vi "myRIO_BRig_RT__Case_Exp_State_SelectPre__v4.vi"(0 "input_dataCurrent":u16[](array[numeric]), 1 "input_SelectWrong":bool, 2 "input_SelectReward":bool, 5 "input_dataExp":u16[](array[numeric]), 7 "input_LickL":bool, 9 "input_LickR":bool, 11 "input_arrTrig":bool[](array[boolean])) -> (3 "output_state":T1, 4 "output_dataCurrent":u16[](array[numeric]), 8 "output_l1_laserEvent":bool, 10 "output_l1_laserOn":bool, 13 "output_l2_laserOn":bool, 14 "output_l2_laserEvent":bool)   [LabVIEW 2014]
uses:
  myRIO_BRig_RT__Case_Exp_stateList.ctl
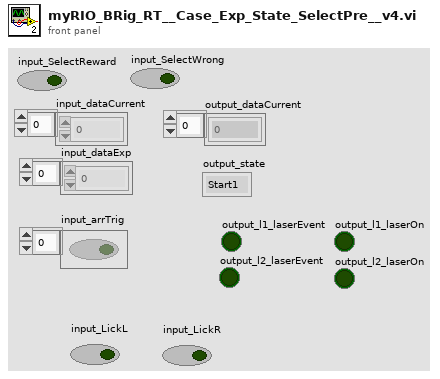
[diagram p1: front panel]
types:
  T1 = typedef "myRIO_BRig_RT__Case_Exp_stateList.ctl" = enum16{"Start1", "Start2", "Start3", "saveSettings1", "saveSettings2", "saveSettings3", "saveSettings4", "saveSettings_LC_ENL_l1", "saveSettings_LC_ENL_l2", "saveSettings_LC_Cue_l1", "saveSettings_LC_Cue_l2", "saveSettings6_LC_l1_Other", "SaveSettings6_LC_l2_Other", "setSettings_Audio", "setSettings_Laser", "initBlock_pre", "initBlock", "initBlock2", "initBlock_post", "initTrial_pre", "initTrial", "initTrial2", "initTrial3", "initTrial4", "initTrial_LC_ENL1", "initTrial_LC_Cue1", "initTrial_LC_Cue1_2", "initTrial_LC_Sel", "initTrial_post", "ENL1_pre", "ENL1", "ENL1_post", "ENL1Penalty_pre", "ENL1Penalty", "ENL2_pre", "ENL2", "ENL2Penalty_pre", "ENL2Penalty", "Cue1_pre", "Cue1", "Cue1_post", "Cue1Penalty_pre", "Cue1Penalty", "Cue2_pre", "Cue2", "Cue2Penalty_pre", "Cue2Penalty", "Selection_pre", "Selection", "Select_post", "SelectReward_pre", "SelectReward", "SelectRewardPost_pre", "SelectRewardPost", "SelectWrong_pre", "SelectWrong", "SelectWrong_post", "SelectTimeout_pre", "SelectTimeout", "SelectTimeout_post", "endTrial_pre", "endTrial1", "endTrial2", "endTrial3", "endTrial_post", "endBlock_pre", "endBlock", "endBlock_post", "endExp", "commConnect", "commUpload_pre", "commUpload_dataBlock", "commUpload_dataCurrent", "commUpload_dataExp", "commUpload_dataLC", "commUpload_dataTrial", "commUpload_post", "saveData_pre", "saveData_dataBlock", "saveData_dataCurrent", "saveData_dataExp", "saveData_dataLC", "saveData_dataTrial", "saveData_post", "empty_endBlock1", "empty_endBlock2", "empty_endTrial1", "empty_endTrial2", "empty_endTrial3", "empty_endTrial4", "empty_endTrial5", "dummyState", "dummyState_endBlock"}
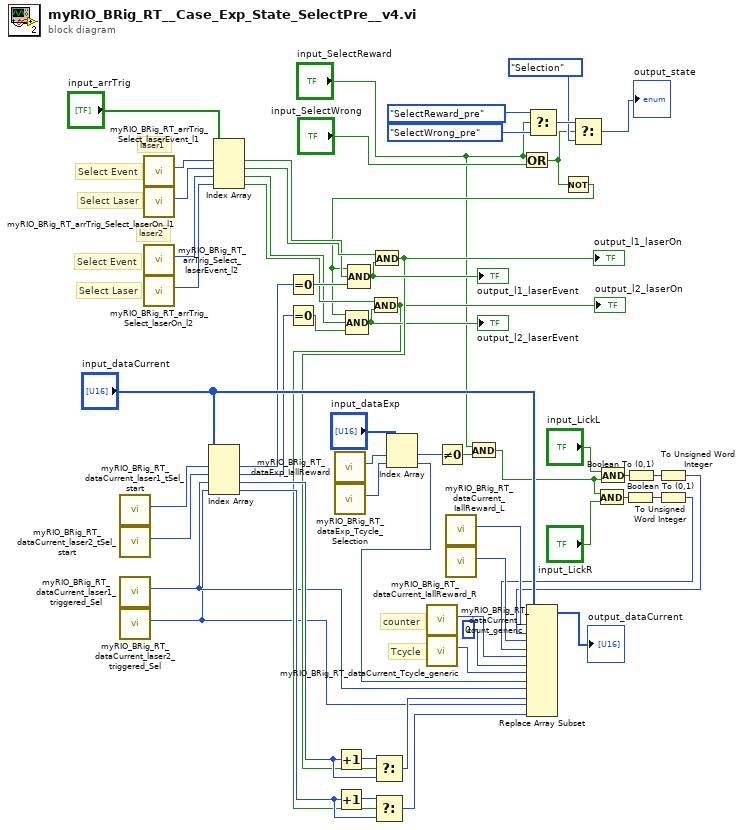
[diagram p0: block diagram]
diagram:
  # "Select Event"
  # "Select Laser"
  # "Select Event"
  # "Select Laser"
  # "laser2"
  # "laser1"
  # "Tcycle"
  # "counter"
  n1 = call "myRIO_BRig_RT_dataCurrent_laser1_tSel_start.vi"() -> ("output_laser1_tSel_start"=w26:i32)  [unwired: 11 in]
  n2 = call "myRIO_BRig_RT_dataCurrent_laser2_tSel_start.vi"() -> ("output_laser2_tSel_start"=w27:i32)  [unwired: 11 in]
  n3 = call "myRIO_BRig_RT_dataCurrent_laser1_triggered_Sel.vi"() -> ("output_laser1_triggered_Selection"=w23:i32)  [unwired: 11 in]
  n4 = call "myRIO_BRig_RT_dataCurrent_laser2_triggered_Sel.vi"() -> ("output_laser2_triggered_Selection"=w22:i32)  [unwired: 11 in]
  n5 = call "myRIO_BRig_RT_arrTrig_Select_laserEvent_l1.vi"() -> ("output_arrTrig_Select_laserEvent_l1"=w41:i32)  [unwired: 11 in]
  n6 = call "myRIO_BRig_RT_arrTrig_Select_laserOn_l1.vi"() -> ("output_arrTrig_Select_laserOn_l1"=w40:i32)  [unwired: 11 in]
  n7 = call "myRIO_BRig_RT_arrTrig_Select_laserEvent_l2.vi"() -> ("output_arrTrig_Select_laserEvent_l2"=w39:i32)  [unwired: 11 in]
  n8 = call "myRIO_BRig_RT_arrTrig_Select_laserOn_l2.vi"() -> ("output_arrTrig_Select_laserOn_l2"=w38:i32)  [unwired: 11 in]
  n9 = Index Array(array="input_dataCurrent", index #1=w26, index #2=w27, index #3=w23, index #4=w22) -> (element #1=w54:u16, element #2=w53:u16, element #3=w50:u16, element #4=w49:u16)
  n10 = Index Array(array="input_arrTrig", index #1=w41, index #2=w40, index #3=w39, index #4=w38) -> (element #1=w33:bool, element #2=w34:bool, element #3=w35:bool, element #4=w36:bool)
  n11 = Equal To 0?(x=w54) -> (x = 0?=w48:bool)
  n12 = Equal To 0?(x=w53) -> (x = 0?=w43:bool)
  n13 = call "myRIO_BRig_RT_dataExp_IallReward.vi"() -> ("output_I_allReward"=w15:i32)  [unwired: 11 in]
  n14 = call "myRIO_BRig_RT_dataExp_Tcycle_Selection.vi"() -> ("output_Tcycle_Selection"=w17:i32)  [unwired: 11 in]
  n15 = Increment(x=w50) -> (x+1=w52:u16)
  n16 = Increment(x=w49) -> (x+1=w51:u16)
  n17 = Index Array(array="input_dataExp", index #1=w15, index #2=w17) -> (element #1=w14:u16, element #2=w16:u16)
  n18 = call "myRIO_BRig_RT_dataCurrent_count_generic.vi"() -> ("output_count_generic"=w57:i32)  [unwired: 11 in]
  n19 = call "myRIO_BRig_RT_dataCurrent_Tcycle_generic.vi"() -> ("output_Tcycle_generic"=w56:i32)  [unwired: 11 in]
  n20 = Not Equal To 0?(x=w14) -> (x != 0?=w13:bool)
  n21 = call "myRIO_BRig_RT_dataCurrent_IallReward_L.vi"() -> ("output_IallReward_L"=w11:i32)  [unwired: 11 in]
  n22 = call "myRIO_BRig_RT_dataCurrent_IallReward_R.vi"() -> ("output_IallReward_R"=w10:i32)  [unwired: 11 in]
  n23 = And(x="input_SelectReward", y=w13) -> (x .and. y?=w9:bool)
  n24 = Or(x="input_SelectReward", y="input_SelectWrong") -> (x .or. y?=w21:bool)
  n25 = Select(t=myRIO_BRig_RT__Case_Exp_stateList."SelectReward_pre" ("Enum"), s="input_SelectReward", f=myRIO_BRig_RT__Case_Exp_stateList."SelectWrong_pre" ("Enum")) -> (s? t:f=w32:T1)
  n26 = Not(x=w21) -> (.not. x?=w20:bool)
  n27 = Compound Arithmetic op=AND(w20, w35, w43) -> (w45:bool)
  "output_l2_laserEvent" <- w45
  n28 = Compound Arithmetic op=AND(w20, w33, w48) -> (w47:bool)
  "output_l1_laserEvent" <- w47
  n29 = And(x=w36, y=w45) -> (x .and. y?=w44:bool)
  "output_l2_laserOn" <- w44
  n30 = And(x=w34, y=w47) -> (x .and. y?=w46:bool)
  "output_l1_laserOn" <- w46
  n31 = Select(t=w52, s=w46, f=w50) -> (s? t:f=w25:u16)
  n32 = Select(t=w51, s=w44, f=w49) -> (s? t:f=w24:u16)
  n33 = Select(t=w32, s=w21, f=myRIO_BRig_RT__Case_Exp_stateList."Selection" ("Enum")) -> (s? t:f=→"output_state":T1)
  n34 = And(x=w9, y="input_LickR") -> (x .and. y?=w5:bool)
  n35 = And(x="input_LickL", y=w9) -> (x .and. y?=w6:bool)
  n36 = Boolean To (0,1)(Boolean=w5) -> (0, 1=w3:i16)
  n37 = Boolean To (0,1)(Boolean=w6) -> (0, 1=w4:i16)
  n38 = To Unsigned Word Integer(number=w4) -> (unsigned 16bit integer=w1:u16)
  n39 = To Unsigned Word Integer(number=w3) -> (unsigned 16bit integer=w2:u16)
  n40 = Replace Array Subset(array="input_dataCurrent", new element #1=w1, index #1=w11, new element #2=w2, index #2=w10, new element #3=u16 0 ("new element/subarray"), index #3=w57, new element #4=w16, index #4=w56, new element #5=w25, index #5=w23, new element #6=w24, index #6=w22) -> (→"output_dataCurrent":u16[])
